vi "DestroyQbus.vi"(8 "error in (no error)":errorcluster, 11 "Qbus":refnum<class "Qbus.lvclass">) -> (0 "error in (no error)":errorcluster)   [LabVIEW 2017, in "Qbus.lvclass"]
doc: "Closes references to queues and to the resources used to implement the Qbus message bus."
uses:
  <vilib>/addons/Qbus/Qbus.lvclass
  <vilib>/addons/Qbus/Qbus.lvclass/Qbus.ctl
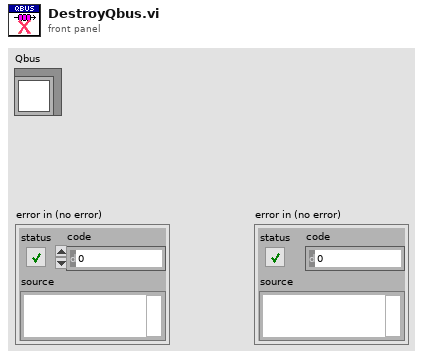
[diagram p1: front panel]
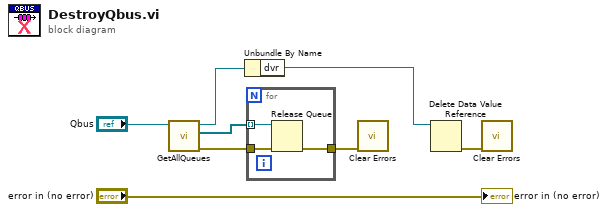
[diagram p0: block diagram]
diagram:
  n1 = call <vilib>:"GetAllQueues.vi"("Qbus in"="Qbus") -> ("error in (no error)"=w8:errorcluster, "queues"=w7:refnum<queue>[], "Qbus out"=w2:refnum<class "Qbus.lvclass">)  [unwired: 8 in]
  n2 = Unbundle By Name(w2) -> ("dvr"=w5:refnum<data-value>)
  n3 = for {
    tunnel: w7 -> [w11] mode=indexing
    tunnel: w8 -> [w10]
    tunnel: [w9] -> w1
    n4 = Release Queue(queue=w11, error in (no error)=w10) -> (error out=w9:errorcluster)  [unwired: 1 in, 2 out]
  }
  n5 = call <vilib>:"Clear Errors.vi"("error in (no error)"=w1) -> ()  [unwired: 5 in, 2 out]
  n6 = Delete Data Value Reference(data value reference=w5) -> (error out=w4:errorcluster)  [unwired: 1 in, 1 out]
  n7 = call <vilib>:"Clear Errors.vi"("error in (no error)"=w4) -> ()  [unwired: 5 in, 2 out]
  "error in (no error)" <- "error in (no error)"
